vi "optionsAcq_zeroFillFactor.vi"(0 "reference":refnum<class "OSA.lvclass">, 2 "zeroFill":u8, 4 "readWrite":enum16{"read", "write"}(ring), 5 "error in (no error)":errorcluster, 7 "ignore range violation (false)":bool) -> (14 "duplicate reference":refnum<class "OSA.lvclass">, 15 "status":string, 16 "zeroFill out":u8, 19 "error out":errorcluster)   [LabVIEW 2010, in "OSA.lvclass"]
uses:
  OSA.lvclass
  OSA20X_misc.lvlib
  FTSLib.dll
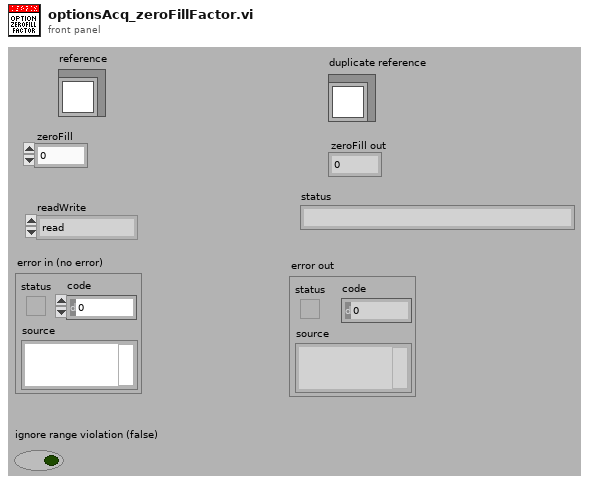
[diagram p1: front panel]
types:
  T1 = typedef "OSA.lvclass/ObjectAttributes.ctl" = cluster{"Stop":bool, "dataType":T2, "spectrometerIdx":u16, "buffer size interferogram":i32, "interferogram":cluster{"new":bool, "plot_x_ min":sgl, "plot_x_max":sgl, "plot_y_min":sgl, "plot_y_max":sgl, "Graph Intrfrgrm":T3, "timeStamp":u32, "signal (%)":dbl, "traces":cluster{"idx":u32, "broadBand":bool, "monoChromatic":bool, "peakToPeakSignal":dbl, "peakToPeakPos":dbl}[], "traces idx last":i32}, "spectrum":cluster{"new":bool, "plot_x_min":sgl, "plot_x_max":sgl, "plot_unit_x":T4, "plot_unit_y":T5, "plot_y_min":sgl, "plot_y_max":sgl, "Graph Spectrum":T3, "timeStamp":u32, "X_VAL_OPTIONS":enum16{"MIN_MAX", "ARRAY"}, "traces":cluster{"idx":u32}[], "traces idx last":i32}, "Thorlabs_OSA_64.lvclass:queue_action.ctlqueue ref":refnum<queue>, "action":T6, "plot zoom step":dbl, "buffer semaphore":T7, "acq stopped":bool, "dataType active":T2, "temperature (degr C)":sgl, "pressure (hPa)":sgl, "rel humidity (%)":sgl, "settings":cluster{"resolution":u16, "sensitivity":u16, "Average":bool, "average nr":u32, "apodisation":T8, "acq delay (ms)":u32, "airMesure":T9, "wmtr on":bool, "intfgrm_smooth_width":u16, "intfgrm_smooth_nrOfPasses":u16, "intfgrm_smooth":T10, "phaseCorrection":T11, "zeroFill":u8, "spectr_smooth":T10, "spectr_smooth_width":u16, "spectr_smooth_nrOfPasses":u16, "resolution (/cm)":sgl, "REF wavelength, (nm)":dbl, "gain_idx":u16, "gainAuto":bool, "gain_relative":dbl, "PD sensitivity mode":T12, "PD senseMode implemented":bool, "SensorTemperature implemented":bool, "SensorPressure implemented":bool, "SensorHumidity implemented":bool, "attenuationAuto":bool, "attenuationOnOff":bool, "attenuationAvailable":bool, "offsetAvailable":bool, "offset":i32, "offset max":u16}, "peaks position":sgl[], "peaks width":sgl[], "peaks height":sgl[], "peaks max nr":u32, "peaks latest nr":i32, "peaks new":bool, "power":dbl, "power new":bool, "path":string, "wavelength (WNr)":dbl, "wavelength new":bool, "buffer size spectrum":i32, "status":string, "vi reference":refnum<vi>, "funcPointer":u64, "libraryPointer":u64, "singleAcquisition":bool, "coherenceLength (cm)":dbl, "coherenceLength new":bool, "spectrometer model":string, "spectrometer serial nr":string, "peaks thld left":sgl[], "peaks thld right":sgl[], "coherenceLength error (cm)":dbl, "ADC bits":u16, "peaks position centroid":sgl[], "peaks height centroid":sgl[], "OSA series":T13, "channel index spectrum":u16, "spectrometer rangeLow, (/cm)":dbl, "spectrometer rangeHigh, (/cm)":dbl, "channel index interferogram":u16, "virtualSource":bool}
  T2 = typedef "OSA.lvclass/acq_dataType.ctl" = enum16{"none", "interferogram", "spectrum"}
  T3 = typedef "OSA.lvclass/graph_intensity.ctl" = refnum<vi>
  T4 = typedef "OSA.lvclass/spectrum_x_unit.ctl" = enum16{"wavenr/cm", "THz", "eV", "nm_air", "nm_vac"}
  T5 = typedef "OSA.lvclass/y_unit.ctl" = enum16{"ADC counts", "dBm pwr absolute", "dBm pwr density", "mW pwr absolute", "mW pwr density"}
  T6 = typedef "OSA.lvclass/queue_action.ctl" = enum16{"none", "stop", "GUI_plotInterferogram", "GUI_plotSpectrum", "GUI_plotInterferogramRescale", "GUI_plotSpectrumRescale", "GUI_plotInterferogramReset", "GUI_plotSpectrumReset", "GUI_plotInterferogramAutoScaleY", "GUI_plotSpectrumAutoScaleY", "GUI_plotInterferogramZoomOut", "GUI_plotSpectrumZoomOut", "GUI_plotInterferogramPane", "GUI_plotSpectrumPane", "GUI_plotInterferogramZoomMouse", "GUI_plotSpectrumZoomMouse", "GUI_spectrumChannelType", "GUI_channel", "ENVIRONMENT temperature", "ENVIRONMENT pressure", "MODE_resolution set", "MODE_resolution get", "MODE_sensitivity set", "MODE_sensitivity get", "MODE_PDTemperature set", "MODE_PDTemperature get", "REBOOT/RESET firmware", "ACQASYNC_acquireSingleSpectrum", "ACQASYNC_continuous start", "ACQASYNC_continuous stop\n", "ACQASYNC_get last interferogram", "ACQASYNC_get last spectrum", "ACQASYNC_get last waveNr", "ACQOPT_interferogram smoothing set", "ACQOPT_interferogram smoothing get", "ACQOPT_spectrum smoothing set", "ACQOPT_spectrum smoothing get", "ACQOPT_apodisation type set", "ACQOPT_apodisation type get", "ACQOPT_phase correction type set", "ACQOPT_phase correction type get", "ACQOPT_acqIntervall_set", "ACQOPT_acqIntervall_get", "ACQOPT_average spectrum set", "ACQOPT_average spectrum get", "ACQOPT_rolling average set", "ACQOPT_rolling average get", "ACQOPT_zero fill factor set", "ACQOPT_zero fill factor get", "ACQOPT_cycle counting set", "ACQOPT_cycle counting get", "ACQOPT_air measure option set", "ACQOPT_air measure option get", "ACQOPT_gainLevel auto get", "ACQOPT_gainLevel auto set", "ACQOPT_gainLevel get", "ACQOPT_gainLevel set", "ACQOPT_offset set", "ACQOPT_attenuator_auto_set", "ACQOPT_attenuator_set", "ACQOPT_getAll", "INSTRUMENT_PROPERTY_range_WaveNr_min", "INSTRUMENT_PROPERTY_range_WaveNr_max", "INSTRUMENT_PROPERTY_reference_wavelength_cm^-1", "INSTRUMENT_PROPERTY_samplesPerRefPeriod", "INSTRUMENT_PROPERTY_resolution_waveNrPercm", "INSTRUMENT_PROPERTY_availableGainLevels", "INSTRUMENT_PROPERTY_status", "CONVERT", "ANALYSE_POWER", "ANALYSE_PEAKS", "ANALYSE_WAVELENGTH", "ANALYSE_SPECTRUM", "ANALYSE_INTERFEROGRAM", "ANALYSE_COHERENCE_LENGTH", "MATH", "MATH_power", "MATH_peaks", "FILE", "miscellaneous"}
  T7 = typedef "Semaphore RefNum" = refnum<k1>
  T8 = typedef "OSA.lvclass/apodisation.ctl" = enum16{"NONE", "NORTON_BEER_WEAK", "NORTON_BEER_MEDIUM", "NORTON_BEER_STRONG", "TRIANGULAR", "COSINE", "HANN", "HAMMING", "BLACKMANHARRIS3", "BLACKMANHARRIS4", "GAUSSIAN"}
  T9 = typedef "OSA.lvclass/airMeasure.ctl" = enum16{"TEMPERATURE", "PRESSURE"}
  T10 = typedef "OSA20X_misc.lvlib/interferogram_smoothing.ctl" = enum16{"NONE", "BINOMIAL", "SAVITSKY_GOLAY", "FOURIER", "MOVING_AVERAGE", "GAUSSIAN"}
  T11 = typedef "OSA.lvclass/phaseCorrection.ctl" = enum16{"NONE", "MERTZ", "FORMAN", "MERTZ_FILE", "FORMAN_FILE", "FUTURE COMP."}
  T12 = typedef "OSA20X_misc.lvlib/PDTemperatureMode.ctl" = enum16{"cool: better sensitivity/noise floor", "warm: extended wl range"}
  T13 = typedef "OSA.lvclass/OSA_series.ctl" = enum16{"OSA200", "OSA300", "UNKNOWN"}
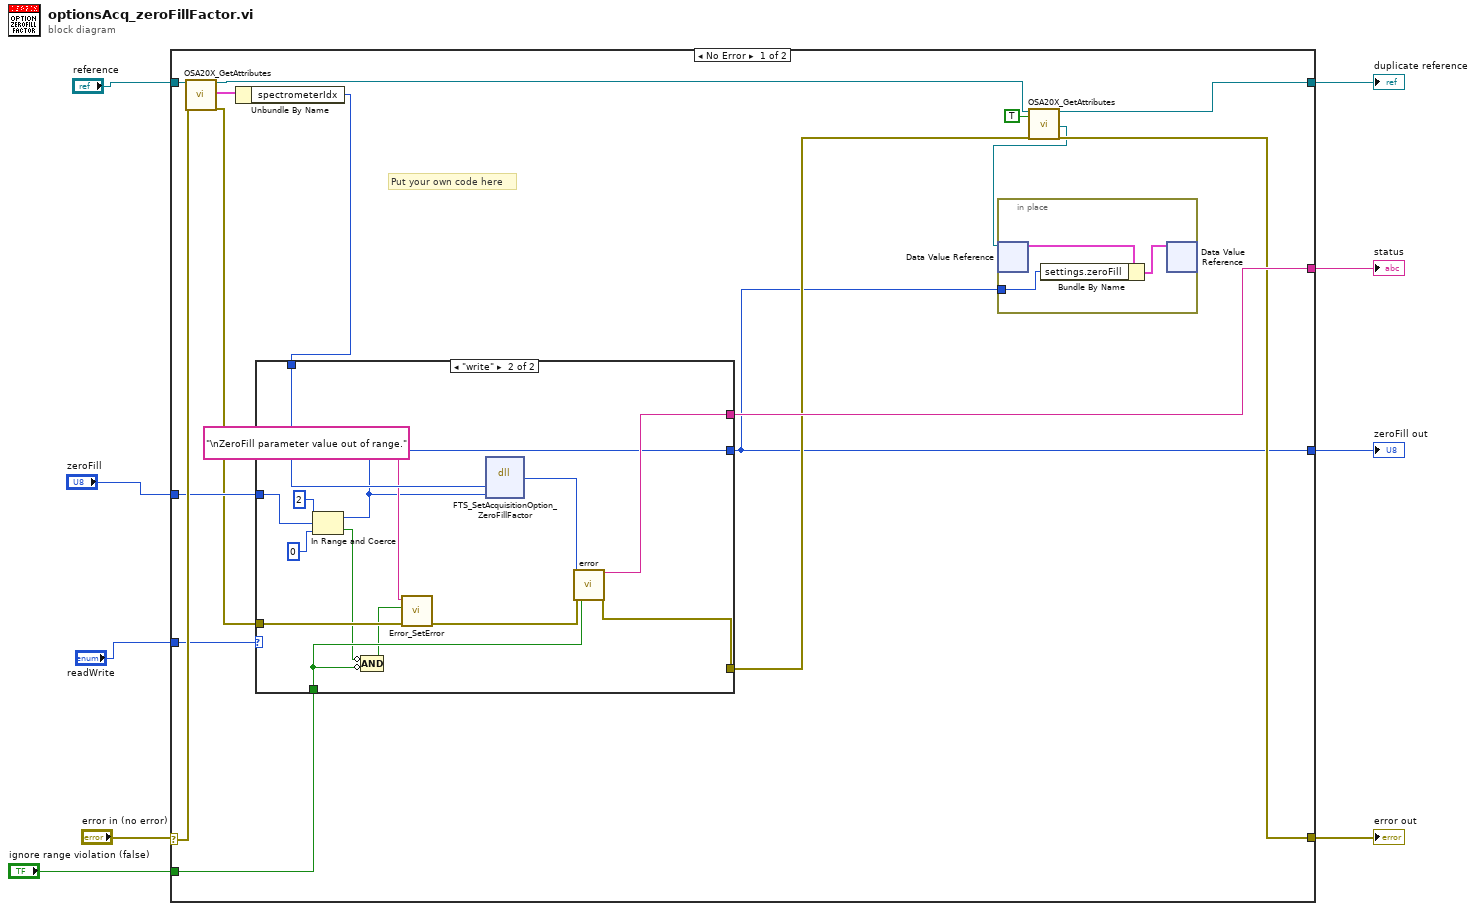
[diagram p0: block diagram]
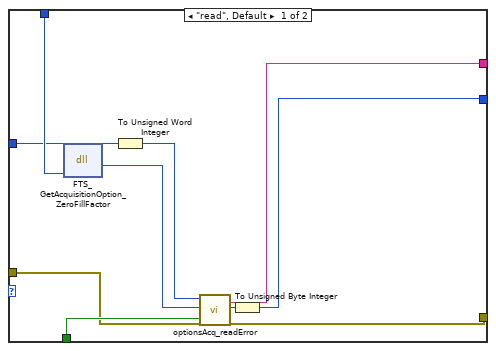
[diagram p2: hidden frame]
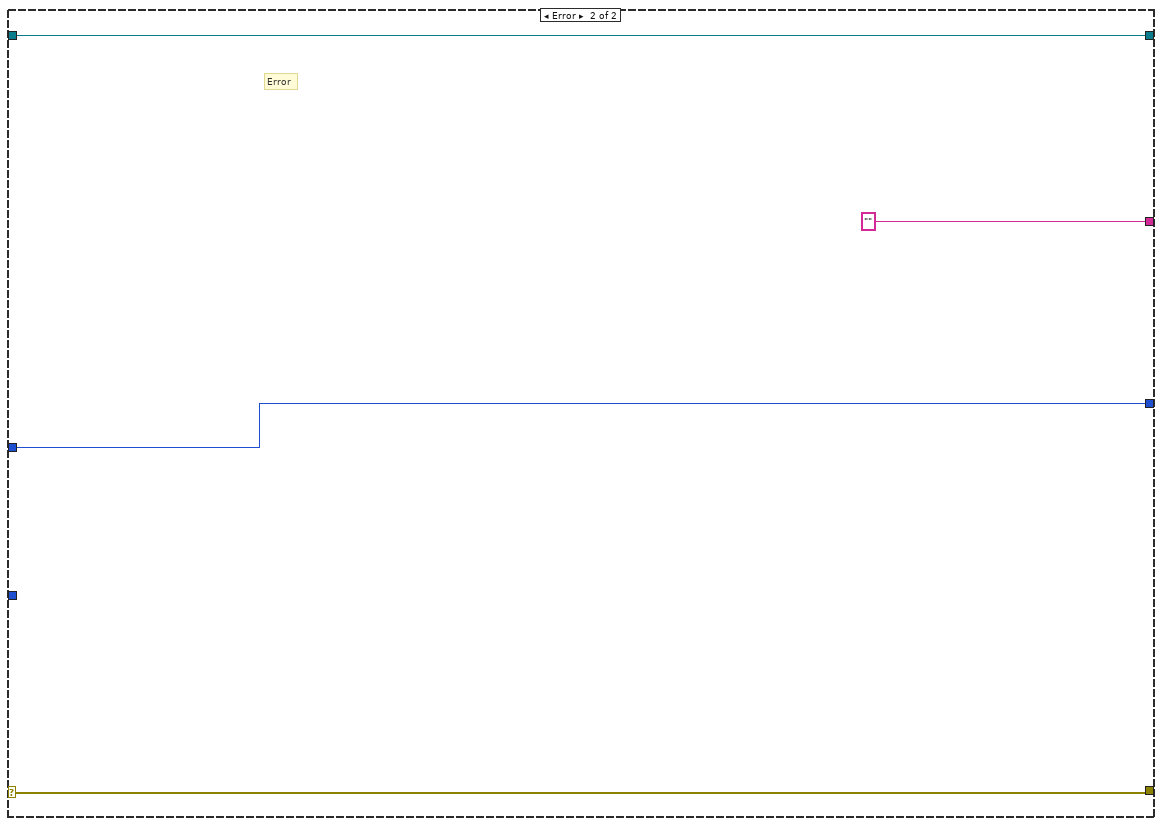
[diagram p3: hidden frame]
diagram:
  n1 = case shown="No Error" "error in (no error)" {
    selector: "error in (no error)" -> [w24 w55]
    tunnel: [w14 w55] -> w9
    tunnel: "reference" -> [w25 w56]
    tunnel: [w17 w56] -> w6
    tunnel: "readWrite" -> [w22 _]
    tunnel: "zeroFill" -> [w19 w53]
    tunnel: [w21 "" ("status")] -> w3
    tunnel: "ignore range violation (false)" -> [w20 _]
    tunnel: [w10 w53] -> w1
    frame No Error {
      # "Put your own code here"
      n2 = call "OSA20X_GetAttributes.vi"("reference in"=w25, "error in (no error)"=w24) -> ("reference out"=w16:refnum<class "OSA.lvclass">, "Data"=w12:T1, "error out"=w18:errorcluster)  [unwired: 14 in, 1 out]
      n3 = Unbundle By Name(w12) -> ("spectrometerIdx"=w23:u16)
      n4 = case shown="\"write\"" w22 {
        tunnel: w23 -> [w38 w52]
        tunnel: w19 -> [w35 w41]
        tunnel: [w34 w50] -> w21
        tunnel: w20 -> [w37 w45]
        tunnel: [w30 w39] -> w10
        tunnel: w18 -> [w31 w47]
        tunnel: [w29 w40] -> w15
        frame "read", Default {
          n5 = dll-call lib="FTSLib.dll" fn="FTS_GetAcquisitionOption_ZeroFillFactor"("spectrIdx"=w38) -> ("return type"=w36:i32)  [unwired: 4 in, 2 out]
          n6 = To Unsigned Word Integer(number=w35) -> (unsigned 16bit integer=w32:u16)
          n7 = call "optionsAcq_readError.vi"("option default"=w32, "option return"=w36, "error in (no error)"=w31, "error ignore"=w37) -> ("status"=w34:string, "option"=w33:u16, "error out"=w29:errorcluster)  [unwired: 13 in]
          n8 = To Unsigned Byte Integer(number=w33) -> (unsigned 8bit integer=w30:u8)
        }
        frame "write" {
          n9 = In Range and Coerce(upper limit=u8 2, x=w41, lower limit=u8 0) -> (coerced(x)=w39:u8, In Range?=w44:bool)
          n10 = Compound Arithmetic op=AND(invert w44, invert w45) -> (w43:bool)
          n11 = call "Error_SetError.vi"("error in"=w47, "status (true)"=w43, "source(\"\")"="\nZeroFill parameter value out of range." ("source(\"\")")) -> ("error out"=w46:errorcluster)  [unwired: 4 in]
          n12 = dll-call lib="FTSLib.dll" fn="FTS_SetAcquisitionOption_ZeroFillFactor"("spectrIdx"=w52, "zeroFillFactor"=w39) -> ("return type"=w51:i32)  [unwired: 5 in, 2 out]
          n13 = call "error.vi"("result code"=w51, "error in (no error)"=w46, "ignore range violation"=w45) -> ("status"=w50:string, "error out"=w40:errorcluster)  [unwired: 14 in, 1 out]
        }
      }
      n14 = call "OSA20X_GetAttributes.vi"("reference in"=w16, "OnlyGetDvrReference(False)"=TRUE, "error in (no error)"=w15) -> ("reference out"=w17:refnum<class "OSA.lvclass">, "DataRef"=w11:refnum<data-value>, "error out"=w14:errorcluster)  [unwired: 13 in, 1 out]
      n15 = in-place {
        in-place-border: w10 -> [w27]
        n16 = in-place-dvr #1(w11) -> (w28:T1)  [unwired: 1 out]
        n17 = Bundle By Name(cluster=w28, "settings.zeroFill"=w27) -> (w26:T1)
        n18 = in-place-dvr #1(w26) -> ()  [unwired: 2 out]
      }
    }
    frame Error {
      # "Error"
    }
  }
  "error out" <- w9
  "duplicate reference" <- w6
  "status" <- w3
  "zeroFill out" <- w1
